vi "Tree Set Time Context.vi"(0 "Tree DVR in":refnum<data-value>, 5 "Start":refnum<data-value>, 7 "End":refnum<data-value>, 9 "Delta":refnum<data-value>, 11 "error in (no error)":errorcluster) -> (4 "Tree DVR out":refnum<data-value>, 15 "error out":errorcluster)   [LabVIEW 2012, in "MDSplus.lvlib"]
doc: "Set the current time context. Only the specified portion of segmented data will be returned by TreeNode.getData() method."
uses:
  <vilib>/MDSplus/Library/MDSplus.lvlib
  <vilib>/MDSplus/Classes/Tree_Class/Tree.lvclass
  <vilib>/MDSplus/Classes/Data_Class/Data.lvclass
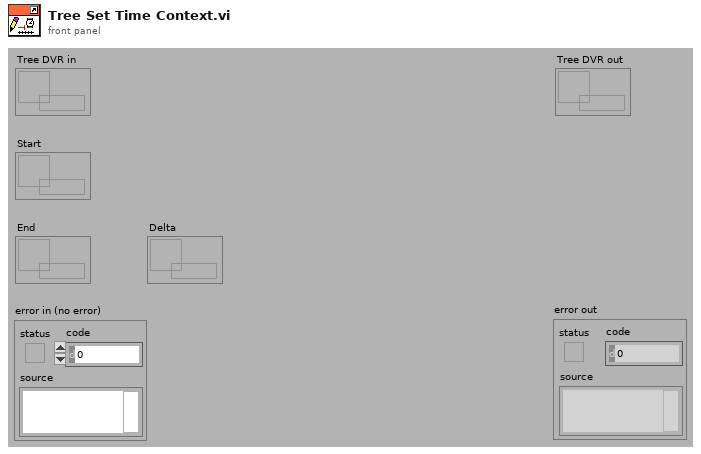
[diagram p1: front panel]
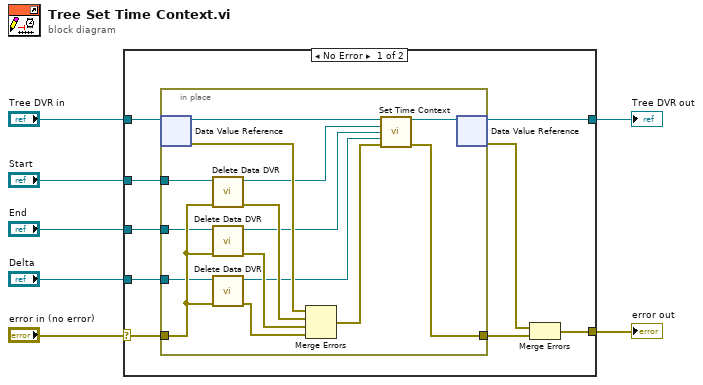
[diagram p0: block diagram]
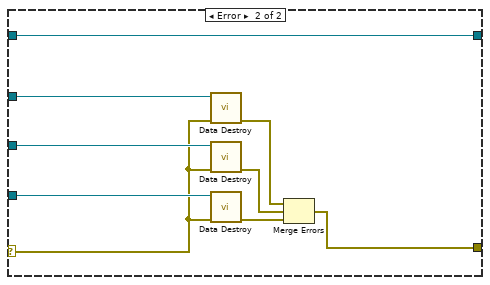
[diagram p2: hidden frame]
diagram:
  n1 = case shown="No Error" "error in (no error)" {
    selector: "error in (no error)" -> [w15 w37]
    tunnel: [w8 w33] -> w7
    tunnel: "Start" -> [w16 w40]
    tunnel: "End" -> [w14 w39]
    tunnel: "Delta" -> [w13 w38]
    tunnel: "Tree DVR in" -> [w12 w32]
    tunnel: [w11 w32] -> w1
    frame No Error {
      n2 = in-place {
        in-place-border: w16 -> [w31]
        in-place-border: w15 -> [w30]
        in-place-border: w14 -> [w29]
        in-place-border: w13 -> [w28]
        in-place-border: [w17] -> w9
        n3 = in-place-dvr #1(w12) -> (w23:refnum<class "Tree.lvclass">, w24:errorcluster)
        n4 = call <vilib>:"Delete Data DVR.vi"("error in (no error)"=w30, "Data DVR in"=w31) -> ("error out"=w25:errorcluster, "Data out"=w21:refnum<class "Data.lvclass">)  [unwired: 8 in]
        n5 = call <vilib>:"Delete Data DVR.vi"("error in (no error)"=w30, "Data DVR in"=w29) -> ("error out"=w26:errorcluster, "Data out"=w20:refnum<class "Data.lvclass">)  [unwired: 8 in]
        n6 = call <vilib>:"Delete Data DVR.vi"("error in (no error)"=w30, "Data DVR in"=w28) -> ("error out"=w27:errorcluster, "Data out"=w19:refnum<class "Data.lvclass">)  [unwired: 8 in]
        n7 = Merge Errors(w24, w25, w26, w27) -> (w22:errorcluster)
        n8 = call-dynamic "Set Time Context.vi"("Tree in"=w23, "Start"=w21, "End"=w20, "Delta"=w19, "error in (no error)"=w22) -> ("Tree out"=w18:refnum<class "Tree.lvclass">, "error out"=w17:errorcluster)  [unwired: 9 in]
        n9 = in-place-dvr #1(w18) -> (w11:refnum<data-value>, w10:errorcluster)
      }
      n10 = Merge Errors(w10, w9) -> (w8:errorcluster)
    }
    frame Error {
      n11 = call <vilib>:"Data Destroy.vi"("error in (no error)"=w37, "Data DVR in"=w40) -> ("error out"=w36:errorcluster)  [unwired: 9 in]
      n12 = call <vilib>:"Data Destroy.vi"("error in (no error)"=w37, "Data DVR in"=w39) -> ("error out"=w35:errorcluster)  [unwired: 9 in]
      n13 = call <vilib>:"Data Destroy.vi"("error in (no error)"=w37, "Data DVR in"=w38) -> ("error out"=w34:errorcluster)  [unwired: 9 in]
      n14 = Merge Errors(w36, w35, w34) -> (w33:errorcluster)
    }
  }
  "error out" <- w7
  "Tree DVR out" <- w1
